vi "CMD_Read Object Command.vi"(11 "value":variant) -> (2 "Command":string, 3 "Object":string)   [LabVIEW 2025]
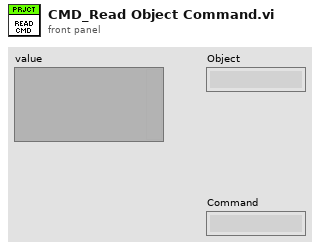
[diagram p1: front panel]
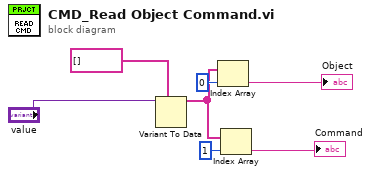
[diagram p0: block diagram]
diagram:
  n1 = Variant To Data(type=string[] [] ("appended array"), Variant="value") -> (data=w3:string[])  [unwired: 1 in, 1 out]
  n2 = Index Array(array=w3, index=0) -> (element=→"Object":string)
  n3 = Index Array(array=w3, index=1) -> (element=→"Command":string)
